vi "XML_Deserialize_XML_File.vi"(8 "error in (no error)":errorcluster, 10 "XSD Path":path, 11 "XML Path":path) -> (0 "error out":errorcluster, 3 "reference out":refnum<k24>)   [LabVIEW 2013, in "XML_Deserializer.lvlib"]
doc: "This VI reads the XML file passed in first argument and validates agains the Schema (.xsd) file passed as second argument.\nIn case if Schema is not validated, an error is returned and some explanation is added to error message."
uses:
  XML_Deserializer.lvlib
  D:/NI/Sales/Canada/Sales/2014/Mon Espace/Modbus Custom-Device/XML Deserializer/XML VIs/API/Sub-VIs/Modbus_CD_XML.dll
  Modbus_CD_XML.dll
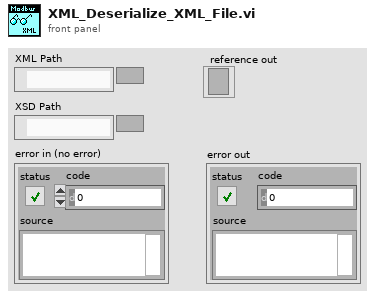
[diagram p1: front panel]
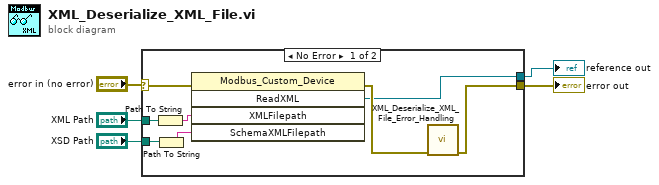
[diagram p0: block diagram]
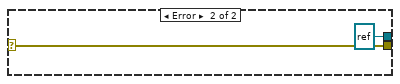
[diagram p2: hidden frame]
diagram:
  n1 = case shown="No Error" "error in (no error)" {
    selector: "error in (no error)" -> [w10 w15]
    tunnel: [w11 w15] -> w5
    tunnel: "XML Path" -> [w13 _]
    tunnel: "XSD Path" -> [w12 _]
    tunnel: [w6 refnum<k24> refnum ("reference out")] -> w1
    frame No Error {
      n2 = Path To String(path=w13) -> (string=w9:string)
      n3 = Path To String(path=w12) -> (string=w8:string)
      n4 = invoke class="Modbus_Custom_Device" method="ReadXML"(error in=w10, "XMLFilepath"=w9, "SchemaXMLFilepath"=w8) -> (error out=w7:errorcluster, "ReadXML"=w6:refnum<k24>)  [unwired: 2 in, 3 out]
      n5 = call "XML_Deserialize_XML_File_Error_Handling.vi"("error in (no error)"=w7) -> ("error out"=w11:errorcluster)  [unwired: 10 in]
    }
    frame Error {
    }
  }
  "error out" <- w5
  "reference out" <- w1
